vi "Read Label (no Class Name).vi"(11 "MSG.lvclass in":refnum<class "MSG.lvclass">) -> (2 "Label":string, 3 "MSG.lvclass out":refnum<class "MSG.lvclass">)   [LabVIEW 2011, in "Messenging.lvlib" / "MSG.lvclass"]
uses:
  MSG.lvclass
  MSG.lvclass/MSG.ctl
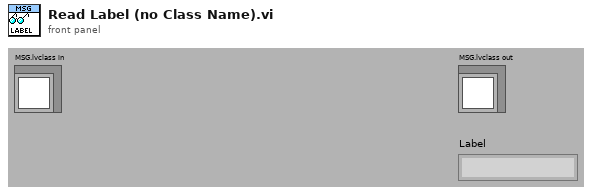
[diagram p1: front panel]
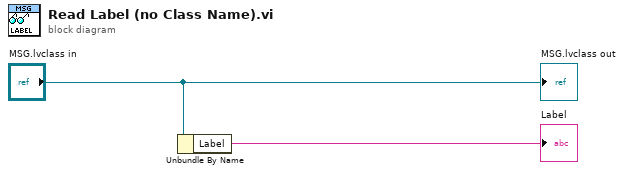
[diagram p0: block diagram]
diagram:
  n1 = Unbundle By Name("MSG.lvclass in") -> ("Label"=→"Label":string)
  "MSG.lvclass out" <- "MSG.lvclass in"
